vi "Data FIFO Probe (U256).vi"(8 "Valid":bool=TRUE, 11 "Data":u64) -> (3 "Array":u64[](array[numeric]))   [LabVIEW 2011]
doc: "This VI is used to probe Array of data on FPGA during simulation"
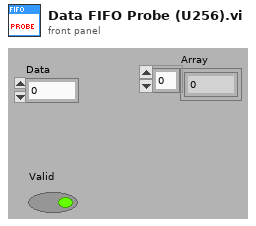
[diagram p1: front panel]
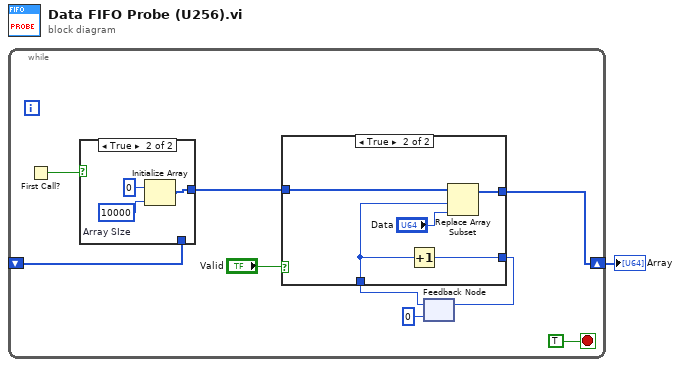
[diagram p0: block diagram]
diagram:
  n1 = while {
    shift-right: [w10] -> w1
    shift-left: _ -> [w8]
    stop <- TRUE stop-if-true
    n2 = First Call?() -> (First Call?: T/F=w6:bool)
    n3 = case shown="True" w6 {
      tunnel: [w18 w19] -> w9
      tunnel: w8 -> [w18 _]
      frame False {
      }
      frame True {
        w21 = 10000  # Array SIze
        n4 = Initialize Array(u64 0 ("element"), w21) -> (w19:u64[])
      }
    }
    n5 = feedback #1(u64 0) -> (w3:u64)
    n6 = case shown="True" "Valid" {
      tunnel: [w12 w17] -> w10
      tunnel: w9 -> [w12 w16]
      tunnel: w3 -> [w11 w14]
      tunnel: [w11 w15] -> w2
      frame False {
      }
      frame True {
        n7 = Increment(x=w14) -> (x+1=w15:u64)
        n8 = Replace Array Subset(array=w16, new element="Data", index=w14) -> (w17:u64[])
      }
    }
    n9 = feedback-in #1(w2) -> ()
  }
  "Array" <- w1
